vi "MigrateLibraryAndOtherfiles.vi"(8 "error in (no error)":errorcluster, 9 "MainModulePath":path, 10 "Project:Open":refnum<vi>, 11 "DependencyList[]":path[](array[path])) -> (0 "error out":errorcluster, 2 "OutsideVIs":string[](array[string]), 3 "DestinationDirectory":path)   [LabVIEW 2021, in "Migrator.lvlib"]
uses:
  Migrator.lvlib
  controls/LibraryData.ctl
  Migrator Reusables/Migrator Reusables.lvlib
  Path Functions/Path Functions.lvlib
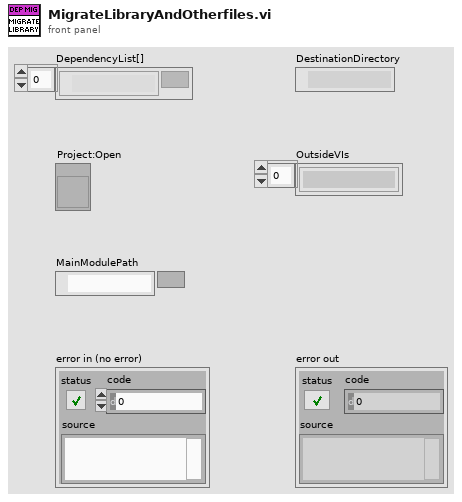
[diagram p1: front panel]
types:
  T1 = typedef "Migrator.lvlib/LibraryData.ctl" = cluster{"LibPath":path, "LibName":string}
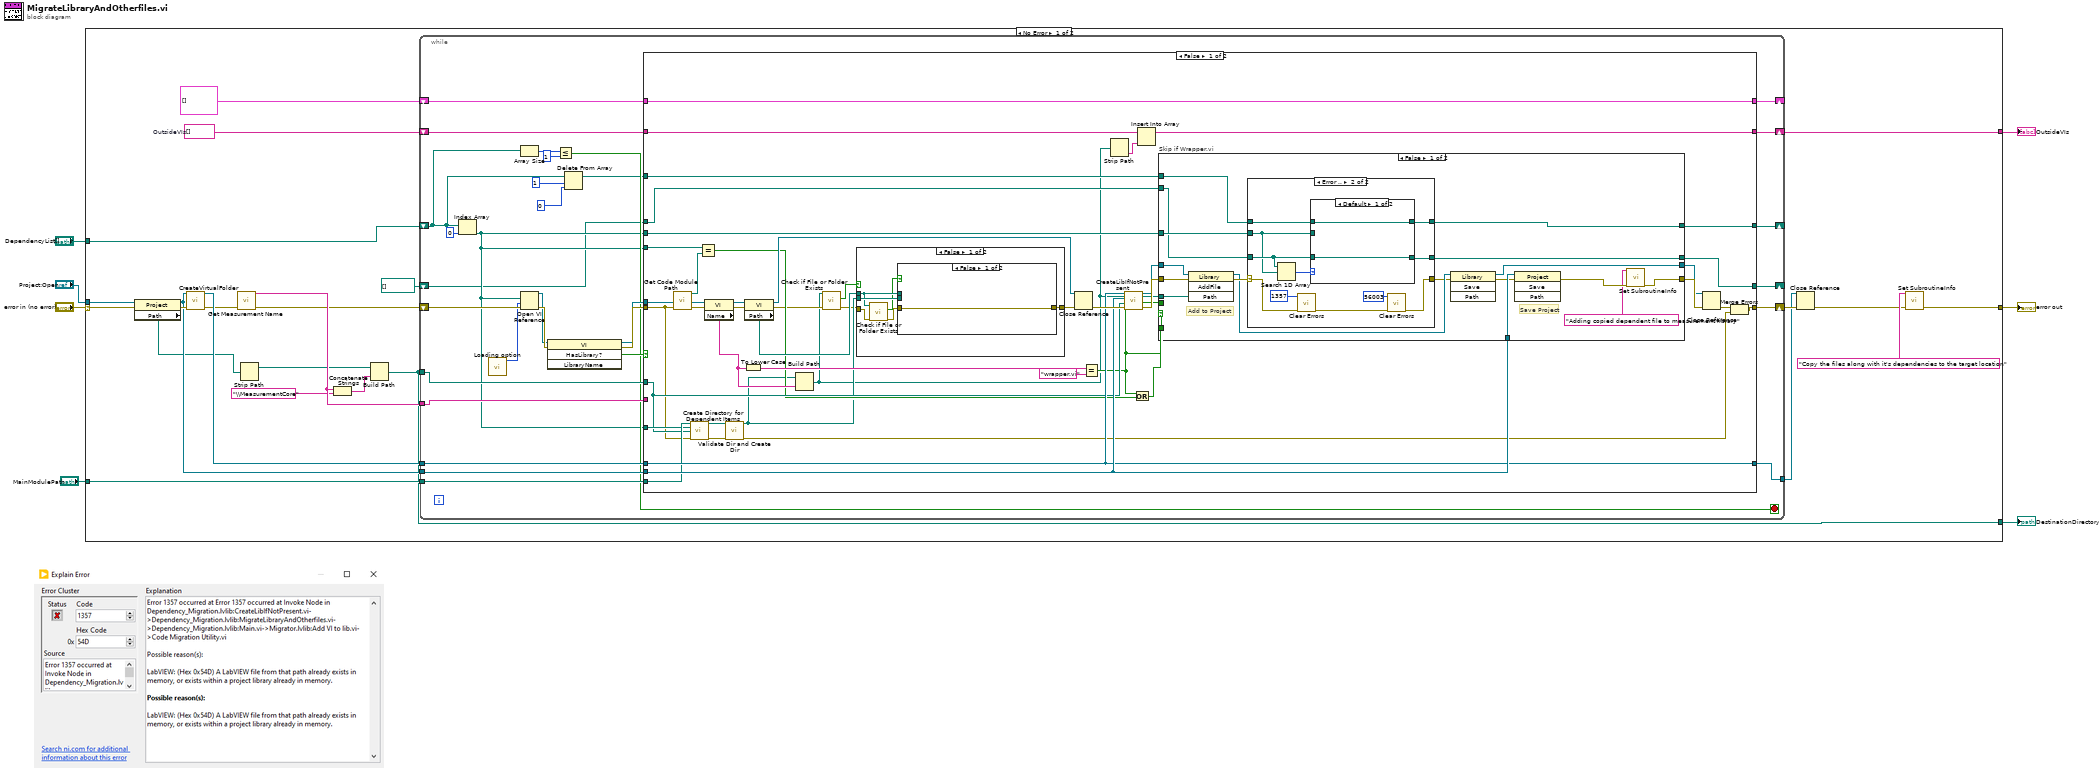
[diagram p0: block diagram]
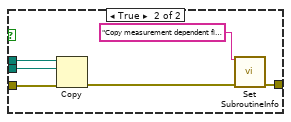
[diagram p2: hidden frame]
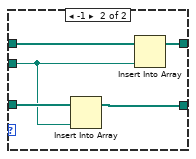
[diagram p5: hidden frame]
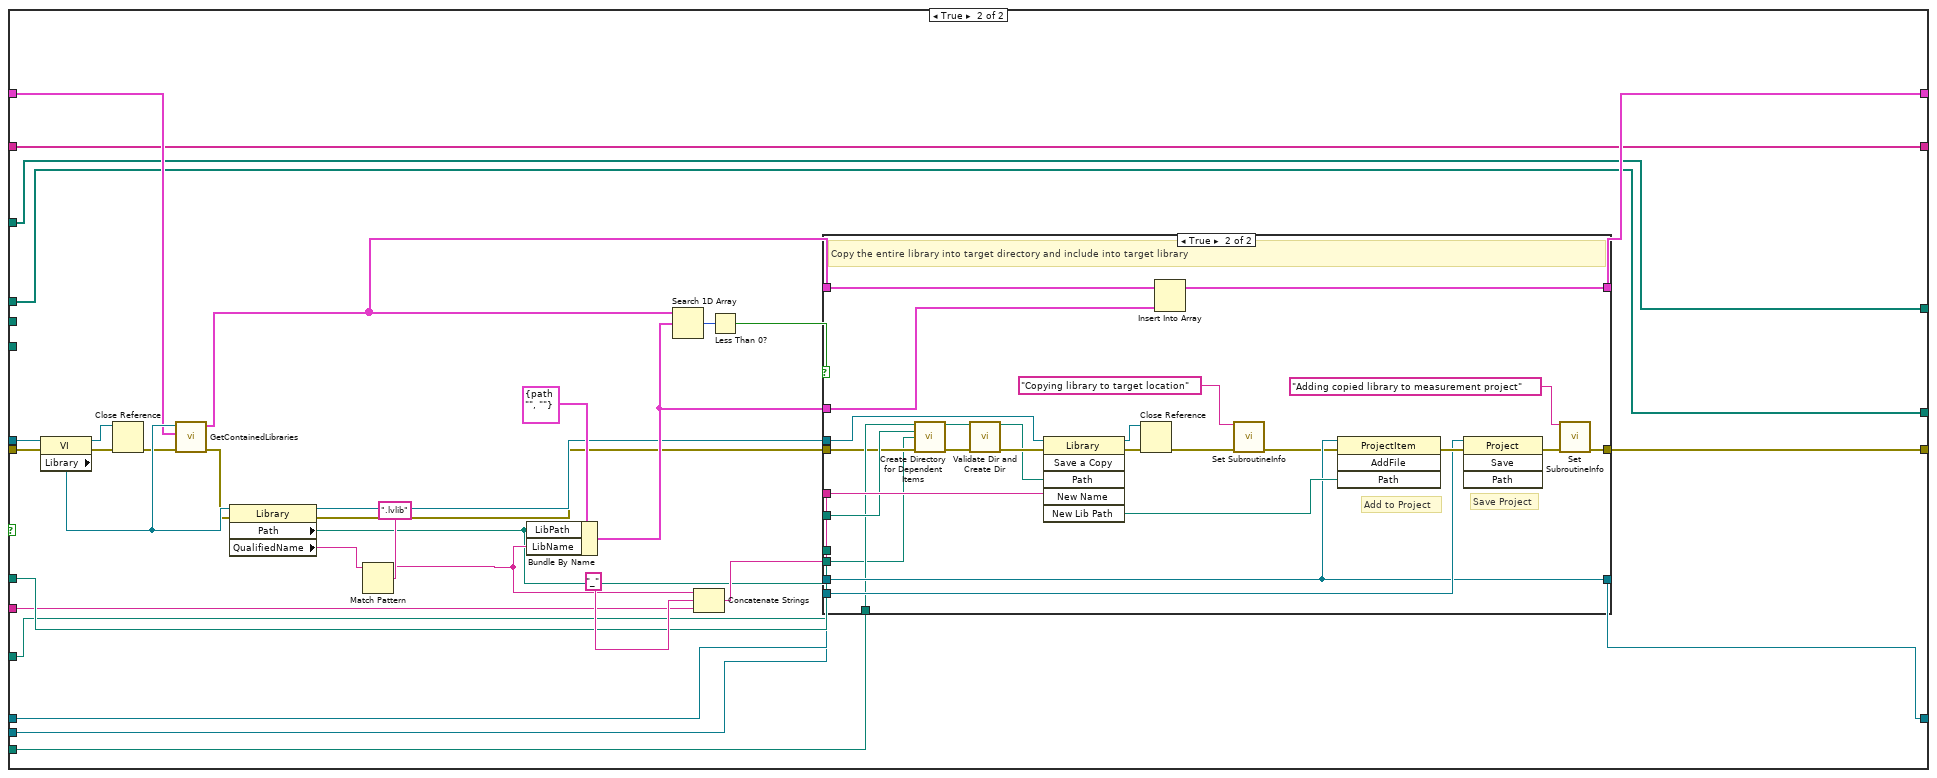
[diagram p7: hidden frame]
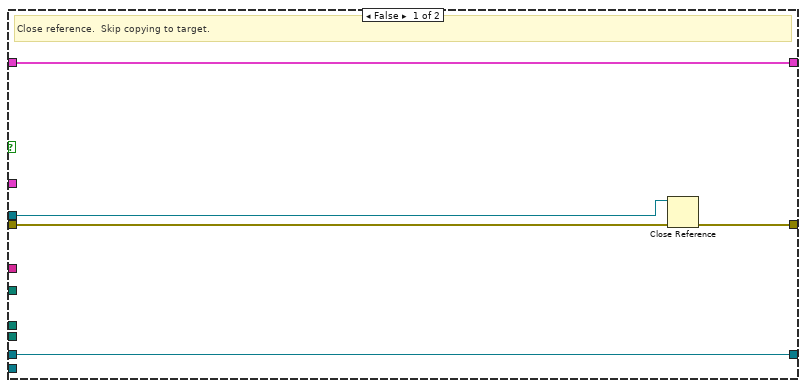
[diagram p8: hidden frame]
diagram:
  n1 = case shown="No Error" "error in (no error)" {
    selector: "error in (no error)" -> [w28 w226]
    tunnel: "Project:Open" -> [w29 _]
    tunnel: [w23 _] -> w5
    tunnel: "MainModulePath" -> [w21 _]
    tunnel: [w15 _] -> w3
    tunnel: "DependencyList[]" -> [w12 _]
    tunnel: [w8 w226] -> w1
    frame No Error {
      w24 = string[] []  # OutsideVIs
      n2 = property class="Project"(reference=w29, error in=w28) -> (reference out=w25:refnum<vi>, error out=w27:errorcluster, "Path"=w20:path)
      n3 = call "CreateVirtualFolder.vi"("error in (no error)"=w27, "Project in"=w25) -> ("error out"=w14:errorcluster, "VirtualFolderRef[]"=w26:refnum<vi>)  [unwired: 8 in]
      n4 = call "Get Measurement Name.vi"("error in (no error)"=w14) -> ("Name Out"=w19:string, "error out"=w13:errorcluster)  [unwired: 13 in]
      n5 = Strip Path(path=w20) -> (stripped path=w16:path)  [unwired: 1 out]
      n6 = Concatenate Strings(w19, "\\MeasurementCore") -> (w17:string)
      n7 = Build Path(base path=w16, name or relative path=w17) -> (appended path=w15:path)
      n8 = while {
        shift-right: [w55] -> _
        shift-left: T1[] [] ("Array") -> [w57]
        tunnel: w26 -> [w52]
        tunnel: w25 -> [w51]
        shift-right: [w49] -> w23
        shift-left: w24 -> [w50]
        tunnel: [w48] -> w22
        tunnel: w21 -> [w47]
        shift-right: [w56] -> w31
        shift-left: w13 -> [w54]
        tunnel: w19 -> [w46]
        tunnel: w15 -> [w45]
        shift-right: [w37] -> _
        shift-left: w12 -> [w41]
        shift-right: [w34] -> _
        shift-left: path[] [] -> [w35]
        stop <- w42 stop-if-true
        n9 = Index Array(array=w41, index=0) -> (element=w36:path)
        n10 = call "Loading option.vi"() -> ("options"=w32:i32)  [unwired: 11 in]
        n11 = Array Size(array=w41) -> (size(s)=w44:i32)
        n12 = Open VI Reference(vi path=w36, options=w32, error in (no error)=w54) -> (vi reference=w59:refnum<vi>, error out=w61:errorcluster)  [unwired: 3 in]
        n13 = invoke class="VI" method="HasLibrary?"(reference=w59, error in=w61) -> (reference out=w58:refnum<vi>, error out=w60:errorcluster, "Has Library?"=w53:bool)  [unwired: 2 in, 1 out]
        n14 = Less Or Equal?(x=w44, y=1) -> (x <= y?=w42:bool)
        n15 = Delete From Array(array=w41, length=1, index=0) -> (array with subset deleted=w38:path[])  [unwired: 1 out]
        n16 = case shown="False" w53 {
          tunnel: w60 -> [w78 w195]
          tunnel: w58 -> [w104 w194]
          tunnel: w45 -> [w79 w176]
          tunnel: w57 -> [w106 w181]
          tunnel: [w81 w186] -> w56
          tunnel: [w106 w185] -> w55
          tunnel: w52 -> [w91 w175]
          tunnel: w51 -> [w93 w174]
          tunnel: w50 -> [w98 w173]
          tunnel: [w97 w173] -> w49
          tunnel: [w91 w172] -> w48
          tunnel: w46 -> [_ w171]
          tunnel: w47 -> [w85 w166]
          tunnel: w36 -> [w84 w165]
          tunnel: w36 -> [w75 _]
          tunnel: w38 -> [w71 w164]
          tunnel: [w70 w164] -> w37
          tunnel: w36 -> [w69 _]
          tunnel: w35 -> [w64 w163]
          tunnel: [w63 w163] -> w34
          frame False {
            n17 = call "Get Code Module Path.vi"("error in (no error)"=w78) -> ("CodeModule Out"=w76:path, "error out"=w77:errorcluster)  [unwired: 13 in]
            n18 = call "Create Directory for Dependent Items.vi"("Old Main Path"=w85, "Old Dependency Path"=w84, "New Dir"=w79, "error in (no error)"=w78) -> ("Directory"=w82:path, "error out"=w83:errorcluster)  [unwired: 10 in]
            n19 = Equal?(x=w75, y=w76) -> (x = y?=w74:bool)
            n20 = property class="VI"(reference=w104, error in=w77) -> (reference out=w103:refnum<vi>, error out=w105:errorcluster, "Name"=w88:string)
            n21 = call "Validate Dir and Create Dir.vi"("Directory"=w82, "error in (no error)"=w83) -> ("Dup Directory"=w68:path, "error out"=w80:errorcluster)  [unwired: 12 in]
            n22 = property class="VI"(reference=w103, error in=w105) -> (reference out=w100:refnum<vi>, error out=w67:errorcluster, "Path"=w101:path)
            n23 = To Lower Case(string=w88) -> (all lower case string=w86:string)
            n24 = Build Path(base path=w68, name or relative path=w88) -> (appended path=w62:path)
            n25 = call <vilib>:"Check if File or Folder Exists.vi"("error in (no error)"=w67, "path"=w62) -> ("error out"=w65:errorcluster, "file or folder exists?"=w66:bool)  [unwired: 7 in, 1 out]
            n26 = case shown="False" w66 {
              tunnel: [w111 w120] -> w102
              tunnel: w101 -> [w110 _]
              tunnel: w68 -> [w112 _]
              tunnel: w65 -> [w109 w120]
              frame False {
                n27 = call <vilib>:"Check if File or Folder Exists.vi"("error in (no error)"=w109, "path"=w110) -> ("error out"=w108:errorcluster, "file or folder exists?"=w107:bool)  [unwired: 7 in, 1 out]
                n28 = case shown="False" w107 {
                  tunnel: w110 -> [_ w119]
                  tunnel: w112 -> [_ w118]
                  tunnel: w108 -> [w113 w117]
                  tunnel: [w113 w114] -> w111
                  frame False {
                  }
                  frame True {
                    n29 = Copy(8:w117, 10:w118, 11:w119) -> (0:w115:errorcluster)  [unwired: 2 in, 2 out]
                    n30 = call "Set SubroutineInfo.vi"("Subroutine In"="Copy measurement dependent file to measurement project location", "error in (no error)"=w115) -> ("error out"=w114:errorcluster)  [unwired: 13 in]
                  }
                }
              }
              frame True {
              }
            }
            n31 = Close Reference(reference=w100, error in (no error)=w102) -> (error out=w95:errorcluster)
            n32 = Equal?(x=w86, y="wrapper.vi") -> (x = y?=w72:bool)
            n33 = Strip Path(path=w62) -> (name=w96:string)  [unwired: 1 out]
            n34 = call "CreateLibIfNotPresent.vi"("error in (no error)"=w95, "DestDirectory"=w79, "ProjectRef"=w93, "VirtualFolderRef"=w91) -> ("error out"=w94:errorcluster, "Library Refnum"=w92:refnum<vi>)  [unwired: 6 in]
            n35 = Or(x=w72, y=w74) -> (x .or. y?=w73:bool)
            n36 = Insert Into Array(array=w98, new element=w96) -> (w97:string[])  [unwired: 1 in]
            n37 = case "Skip if Wrapper.vi" shown="False" w72 {
              tunnel: [w122 w162] -> w99
              tunnel: w62 -> [w136 _]
              tunnel: w94 -> [w135 w162]
              tunnel: w93 -> [w134 _]
              tunnel: w92 -> [w133 w161]
              tunnel: [w131 w161] -> w89
              tunnel: w72 -> [_ _]
              tunnel: w73 -> [_ _]
              tunnel: w71 -> [w128 w160]
              tunnel: [w127 w160] -> w70
              tunnel: w69 -> [w126 _]
              tunnel: w64 -> [w125 w159]
              tunnel: [w124 w159] -> w63
              frame False {
                # "Save Project"
                # "Add to Project"
                n38 = invoke class="Library" method="AddFile"(reference=w133, error in=w135, "Path"=w136) -> (reference out=w132:refnum<vi>, error out=w137:errorcluster)  [unwired: 1 in, 2 out]
                n39 = case shown="Error .." w137 {
                  selector: w137 -> [w139 w151]
                  tunnel: [w139 w147] -> w129
                  tunnel: w128 -> [w140 w146]
                  tunnel: [w140 w145] -> w127
                  tunnel: w126 -> [_ w142]
                  tunnel: w125 -> [w138 w143]
                  tunnel: [w138 w144] -> w124
                  frame No Error {
                  }
                  frame Error {
                    n40 = Search 1D Array(1D array=w143, element=w142) -> (index of element=w141:i32)  [unwired: 1 in]
                    n41 = call <vilib>:"Clear Errors.vi"("error in (no error)"=w151, "specific error code to clear (0: all)"=1357) -> ("error out"=w148:errorcluster)  [unwired: 4 in, 1 out]
                    n42 = case shown="Default" w141 {
                      tunnel: w146 -> [w153 w158]
                      tunnel: [w153 w157] -> w145
                      tunnel: [w152 w156] -> w144
                      tunnel: w143 -> [w152 w155]
                      tunnel: w142 -> [_ w154]
                      frame Default {
                      }
                      frame -1 {
                        n43 = Insert Into Array(array=w155, new element=w154) -> (w156:path[])  [unwired: 1 in]
                        n44 = Insert Into Array(array=w158, new element=w154) -> (w157:path[])  [unwired: 1 in]
                      }
                    }
                    n45 = call <vilib>:"Clear Errors.vi"("error in (no error)"=w148, "specific error code to clear (0: all)"=56003) -> ("error out"=w147:errorcluster)  [unwired: 4 in, 1 out]
                  }
                }
                n46 = invoke class="Library" method="Save"(reference=w132, error in=w129) -> (reference out=w131:refnum<vi>, error out=w130:errorcluster)  [unwired: 2 in, 2 out]
                n47 = invoke class="Project" method="Save"(reference=w134, error in=w130) -> (error out=w123:errorcluster)  [unwired: 2 in, 3 out]
                n48 = call "Set SubroutineInfo.vi"("Subroutine In"="Adding copied dependent file to measurement library", "error in (no error)"=w123) -> ("error out"=w122:errorcluster)  [unwired: 13 in]
              }
              frame True {
              }
            }
            n49 = Close Reference(reference=w89, error in (no error)=w99) -> (error out=w90:errorcluster)
            n50 = Merge Errors(w90, w80) -> (w81:errorcluster)
          }
          frame True {
            n51 = property class="VI"(reference=w194, error in=w195) -> (reference out=w184:refnum<vi>, error out=w193:errorcluster, "Library"=w183:refnum<vi>)
            n52 = Close Reference(reference=w184, error in (no error)=w193) -> (error out=w180:errorcluster)
            n53 = call "GetContainedLibraries.vi"("error in (no error)"=w180, "LibDataIn[]"=w181, "Library in"=w183) -> ("error out"=w179:errorcluster, "LibDataOut[]"=w182:T1[])  [unwired: 7 in]
            n54 = property class="Library"(reference=w183, error in=w179) -> (reference out=w188:refnum<vi>, error out=w187:errorcluster, "Path"=w167:path, "QualifiedName"=w169:string)
            n55 = Match Pattern(string=w169, regular expression=".lvlib") -> (before substring=w168:string)  [unwired: 1 in, 3 out]
            n56 = Bundle By Name(cluster=T1 {"LibPath"=path "", "LibName"=""}, "LibPath"=w167, "LibName"=w168) -> (w189:T1)
            n57 = Search 1D Array(1D array=w182, element=w189) -> (index of element=w191:i32)  [unwired: 1 in]
            n58 = Concatenate Strings(w168, "_" ("string"), w171) -> (w178:string)
            n59 = Less Than 0?(x=w191) -> (x < 0?=w190:bool)
            n60 = case shown="True" w190 {
              tunnel: w189 -> [_ w223]
              tunnel: w182 -> [w200 w224]
              tunnel: [w200 w225] -> w185
              tunnel: w187 -> [w197 w210]
              tunnel: w188 -> [w198 w222]
              tunnel: [w199 w205] -> w186
              tunnel: w176 -> [_ w207]
              tunnel: w178 -> [_ w218]
              tunnel: w175 -> [w196 w215]
              tunnel: w174 -> [_ w216]
              tunnel: [w196 w215] -> w172
              tunnel: w167 -> [_ w214]
              tunnel: w166 -> [_ w213]
              tunnel: w165 -> [_ _]
              frame False {
                # "Close reference.  Skip copying to target."
                n61 = Close Reference(reference=w198, error in (no error)=w197) -> (error out=w199:errorcluster)
              }
              frame True {
                # "Save Project"
                # "Add to Project"
                # "Copy the entire library into target directory and include into target library"
                n62 = call "Create Directory for Dependent Items.vi"("Old Main Path"=w213, "Old Dependency Path"=w214, "New Dir"=w207, "error in (no error)"=w210) -> ("Directory"=w212:path, "error out"=w211:errorcluster)  [unwired: 10 in]
                n63 = call "Validate Dir and Create Dir.vi"("Directory"=w212, "error in (no error)"=w211) -> ("Dup Directory"=w208:path, "error out"=w209:errorcluster)  [unwired: 12 in]
                n64 = invoke class="Library" method="Save a Copy"(reference=w222, error in=w209, "Path"=w208, "New Name"=w218) -> (reference out=w219:refnum<vi>, error out=w220:errorcluster, "New Lib Path"=w217:path)  [unwired: 2 in, 3 out]
                n65 = Close Reference(reference=w219, error in (no error)=w220) -> (error out=w203:errorcluster)
                n66 = Insert Into Array(array=w224, new element=w223) -> (w225:T1[])  [unwired: 1 in]
                n67 = call "Set SubroutineInfo.vi"("Subroutine In"="Copying library to target location", "error in (no error)"=w203) -> ("error out"=w202:errorcluster)  [unwired: 13 in]
                n68 = invoke class="ProjectItem" method="AddFile"(reference=w215, error in=w202, "Path"=w217) -> (error out=w221:errorcluster)  [unwired: 1 in, 3 out]
                n69 = invoke class="Project" method="Save"(reference=w216, error in=w221) -> (error out=w206:errorcluster)  [unwired: 2 in, 3 out]
                n70 = call "Set SubroutineInfo.vi"("Subroutine In"="Adding copied library to measurement project", "error in (no error)"=w206) -> ("error out"=w205:errorcluster)  [unwired: 13 in]
              }
            }
          }
        }
      }
      n71 = Close Reference(reference=w22, error in (no error)=w31) -> (error out=w9:errorcluster)
      n72 = call "Set SubroutineInfo.vi"("Subroutine In"="Copy the files along with it's dependencies to the target location", "error in (no error)"=w9) -> ("error out"=w8:errorcluster)  [unwired: 13 in]
    }
    frame Error {
    }
  }
  "error out" <- w1
  "DestinationDirectory" <- w3
  "OutsideVIs" <- w5
